vi "Apply Transparency.vi"(9 "Rect (32,32)":T1={"left"=0, "top"=0, "right"=32, "bottom"=32}, 10 "depth (24)":i32=24, 11 "Pic In":picture) -> (3 "image data":T2={"image type"=0, "image depth"=0, "image"=array[4096 elements], "mask"=[], "colors"=[], "Rectangle"={"left"=0, "top"=0, "right"=32, "bottom"=32}})   [LabVIEW 2020, in "LabVIEW Icon API.lvlib"]
doc: "Apply transparency on a glyph."
uses:
  LabVIEW Icon API.lvlib
  lv_icon/lv_icon.lvlib
  <vilib>/picture/picture.llb/imagedata.ctl
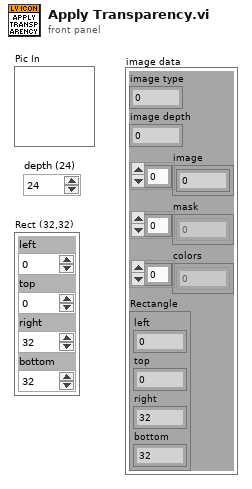
[diagram p1: front panel]
types:
  T1 = cluster{"left":i16, "top":i16, "right":i16, "bottom":i16}
  T2 = typedef "imagedata.ctl" = cluster{"image type":i32, "image depth":i32, "image":u8[], "mask":u8[], "colors":u32[], "Rectangle":cluster{"left":i16, "top":i16, "right":i16, "bottom":i16}}
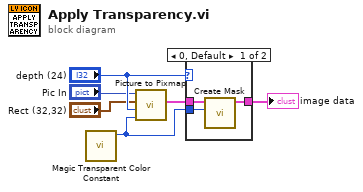
[diagram p0: block diagram]
diagram:
  n1 = call "Magic Transparent Color Constant.vi"() -> ("Magic transparent color constant"=w6:u32)  [unwired: 11 out]
  n2 = call <vilib>:"Picture to Pixmap.vi"("Background Color"=w6, "depth"="depth (24)", "rect"="Rect (32,32)", "picture"="Pic In") -> ("image data"=w2:T2)  [unwired: 7 out]
  n3 = case shown="0, Default" "depth (24)" {
    tunnel: w2 -> [w9 w10]
    tunnel: w6 -> [w8 _]
    tunnel: [w7 w10] -> w4
    frame 0, Default {
      n4 = call <vilib>:"Create Mask.vi"("Mask Color (Black)"=w8, "image data"=w9) -> ("image data"=w7:T2)  [unwired: 2 in, 7 out]
    }
    frame 1 {
    }
  }
  "image data" <- w4
